vi "Init.vi"(8 "error in (no error)":errorcluster, 10 "Frames":u16, 11 "Millis":u16) -> (0 "error out":errorcluster, 3 "Sleep out":refnum<class "Sleep.lvclass">)   [LabVIEW 2022 SP3, in "obs-websocket-lv.lvlib" / "Sleep.lvclass"]
uses:
  Sleep.lvclass
  Sleep.lvclass/Sleep.ctl
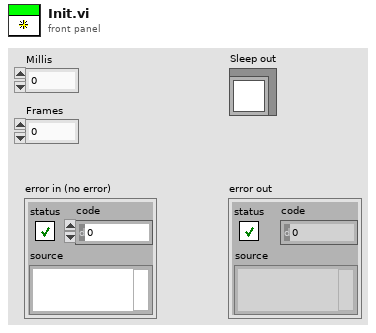
[diagram p1: front panel]
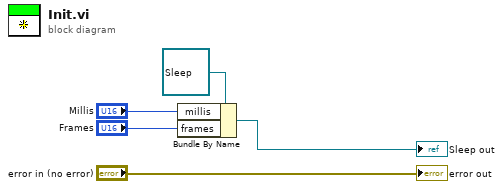
[diagram p0: block diagram]
diagram:
  n1 = Bundle By Name(cluster=refnum<class "Sleep.lvclass"> refnum ("Sleep in"), "millis"="Millis", "frames"="Frames") -> (→"Sleep out":refnum<class "Sleep.lvclass">)
  "error out" <- "error in (no error)"
